vi "DeleteBlockData.vi"(10 "Block Data In":T1) -> (2 "Block Data Out":T1)   [LabVIEW 2013]
uses:
  BlockData.ctl
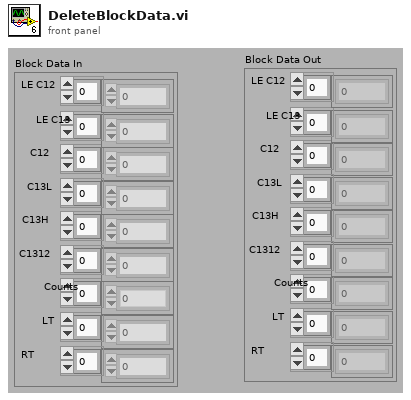
[diagram p1: front panel]
types:
  T1 = typedef "BlockData.ctl" = cluster{"LE C12":dbl[], "LE C13":dbl[], "C12":dbl[], "C13L":dbl[], "C13H":dbl[], "C1312":dbl[], "Counts":u32[], "LT":dbl[], "RT":dbl[]}
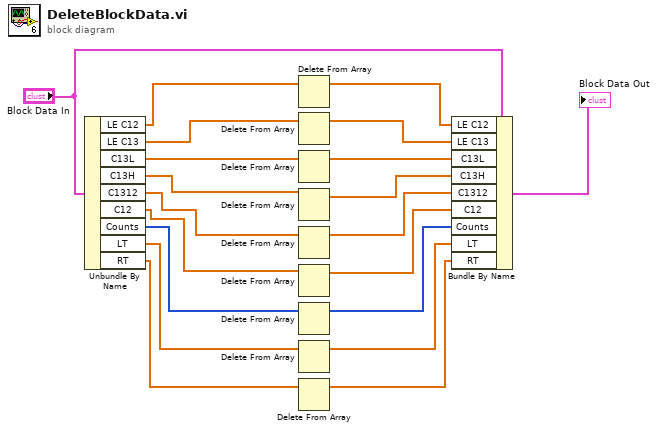
[diagram p0: block diagram]
diagram:
  n1 = Unbundle By Name("Block Data In") -> ("LE C12"=w2:dbl[], "LE C13"=w4:dbl[], "C13L"=w10:dbl[], "C13H"=w7:dbl[], "C1312"=w9:dbl[], "C12"=w8:dbl[], "Counts"=w20:u32[], "LT"=w19:dbl[], "RT"=w18:dbl[])
  n2 = Delete From Array(array=w2) -> (array with subset deleted=w1:dbl[])  [unwired: 2 in, 1 out]
  n3 = Delete From Array(array=w4) -> (array with subset deleted=w3:dbl[])  [unwired: 2 in, 1 out]
  n4 = Delete From Array(array=w10) -> (array with subset deleted=w11:dbl[])  [unwired: 2 in, 1 out]
  n5 = Delete From Array(array=w7) -> (array with subset deleted=w12:dbl[])  [unwired: 2 in, 1 out]
  n6 = Delete From Array(array=w9) -> (array with subset deleted=w13:dbl[])  [unwired: 2 in, 1 out]
  n7 = Delete From Array(array=w8) -> (array with subset deleted=w14:dbl[])  [unwired: 2 in, 1 out]
  n8 = Delete From Array(array=w20) -> (array with subset deleted=w17:u32[])  [unwired: 2 in, 1 out]
  n9 = Delete From Array(array=w19) -> (array with subset deleted=w16:dbl[])  [unwired: 2 in, 1 out]
  n10 = Delete From Array(array=w18) -> (array with subset deleted=w15:dbl[])  [unwired: 2 in, 1 out]
  n11 = Bundle By Name(cluster="Block Data In", "LE C12"=w1, "LE C13"=w3, "C13L"=w11, "C13H"=w12, "C1312"=w13, "C12"=w14, "Counts"=w17, "LT"=w16, "RT"=w15) -> (→"Block Data Out":T1)
